vi "x502_recv.vi"() -> ()   [LabVIEW 2010]
uses:
  <vilib>/Waveform/DWDTOps.llb/DWDT Binary U32 to Digital.vi
panel:
  in  "Подключение по IP":bool
  in  "IP Addr":string="192.168.0.1"
  out "MCU ver":string
  in  "START":bool
  in  "Список устройств USB/PCIe":u16(ring) items=["L502, 111"]
  out "Mixed Signal Graph":T1(graph)
  in  "Логические каналы":T2(array[cluster])=[{"PhyCh"=1, "Avg"=1, "Mode"=1, "Range"=0}, {"PhyCh"=2, "Avg"=1, "Mode"=1, "Range"=0}, {"PhyCh"=3, "Avg"=1, "Mode"=1, "Range"=0}] {"Range" items=["10 В", "5 В", "2 В", "1 В", "0.5 В", "0.2 В"]; "Mode" items=["С общей землей", "Дифференциальный", "Измерение нуля"]; "Avg" max=255 step=1; "PhyCh" min=1 max=32 step=1}
  in  "Отображать за время":dbl=250.0 min=10.0 step=1.0
  in  "stop":bool
  out "Установленная частота синхронного ввода DIN":dbl=2.0 min=2.0 max=2000000.0 format="%#_8f"
  in  "Частота синхронного ввода DIN":dbl=20000.0 min=1.0 max=2000000.0 format="%#_8f"
  out "FPGA Ver":string
  in  "Количество каналов":u32=3 min=1 max=3
  out "Установленная частота на канал":dbl=2.0 min=2.0 max=2000000.0 format="%#_8f"
  out "Установленная частота сбора":dbl=2.0 min=2.0 max=2000000.0 format="%#_8f"
  in  "Частота сбора на канал":dbl=2000000.0 min=2.0 max=2000000.0 format="%#_8f"
  in  "Частота сбора (Гц)":dbl=2000000.0 min=2.0 max=2000000.0 format="%#_8f"
  out "PldaVer":u8
  out "Serial":string
  out "Name":string
  # "Информация о плате"
  # "Настройки модуля"
  # "Устанавливаемое"
  # "Установленное"
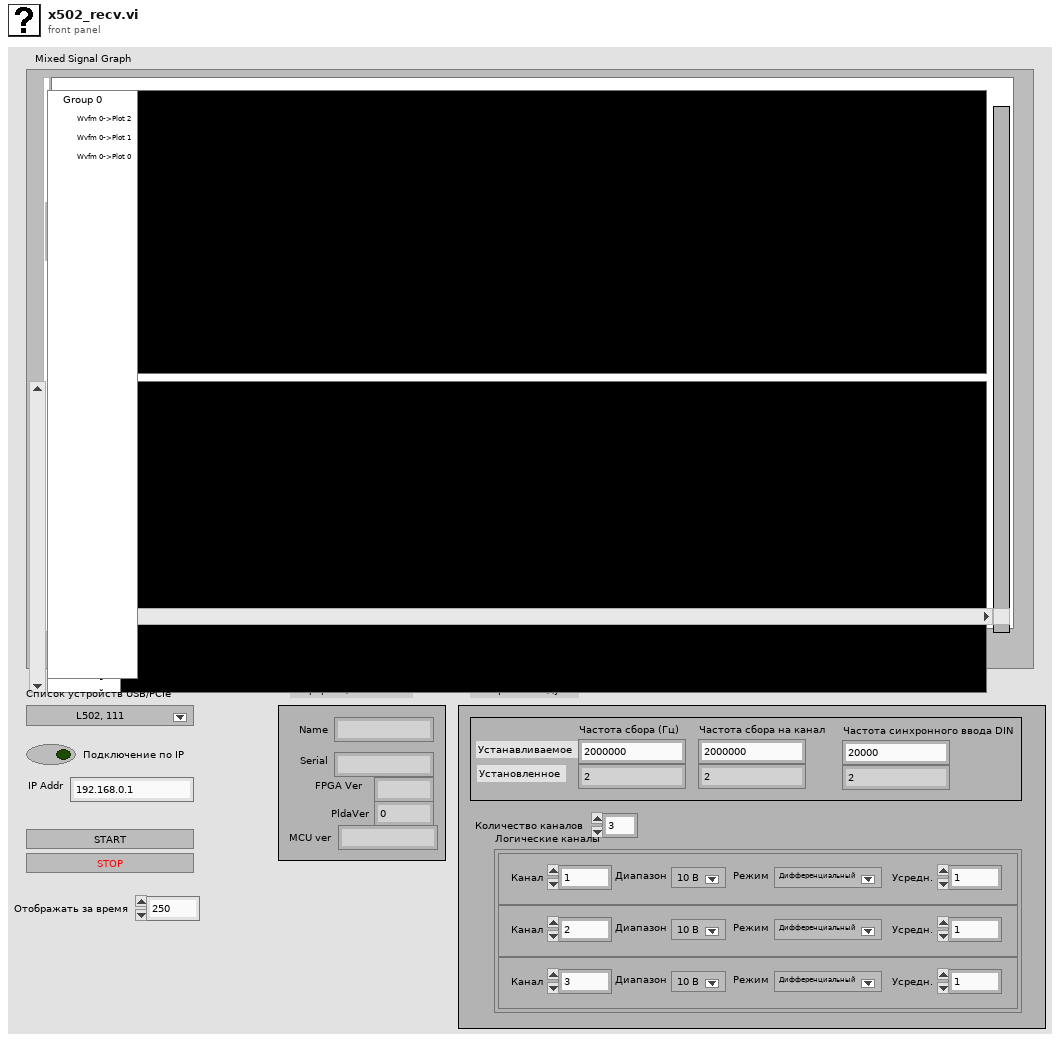
[diagram p1: front panel]
types:
  T1 = cluster{"Dynamic Data Type":dynamicdata, "digital waveform":digitalwaveform}
  T2 = cluster{"PhyCh":u32, "Avg":u32, "Mode":u32, "Range":u32}[]
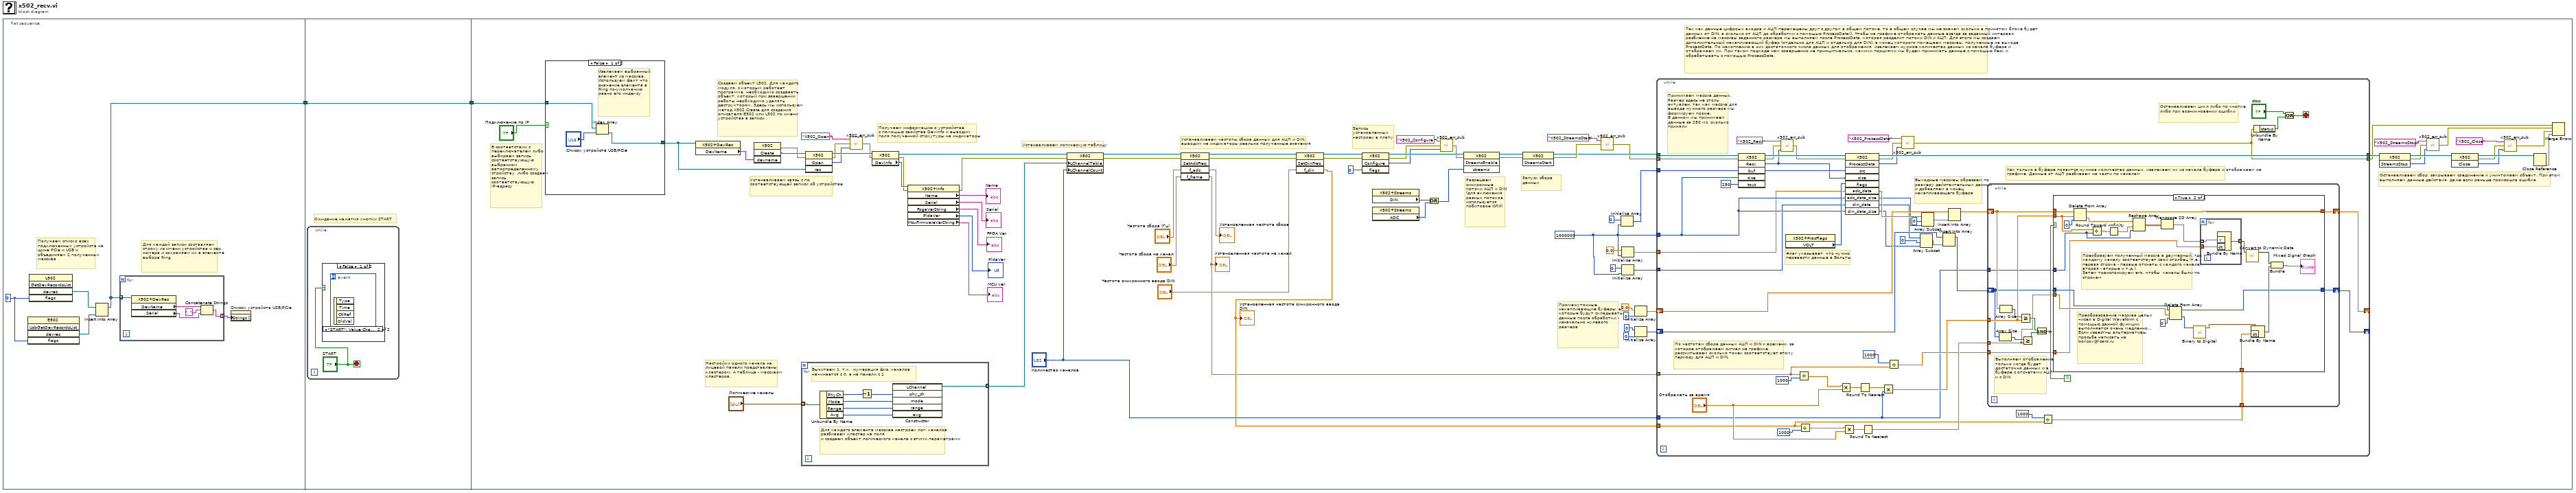
[diagram p0: block diagram]
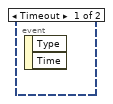
[diagram p2: hidden frame]
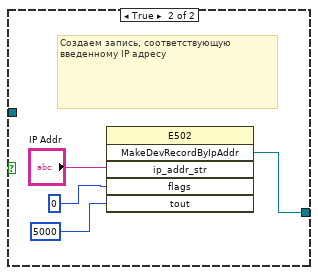
[diagram p4: hidden frame]
diagram:
  n1 = flat-sequence {
    tunnel: [w3] -> w1
    tunnel: [w13] -> w2
    tunnel: w1 -> [w13]
    tunnel: w2 -> [w21]
    frame #0 {
      w5 = 0
      # "Для каждой записи составляем строку из имени устройства и сер. номера и сохраняем их в элементе выбора Ring"
      # "Получаем списко всех подключенных устройств на шине PCIe и USB и объединяем 2 полученных массива"
      n2 = invoke class="E502" method="UsbGetDevRecordsList"("flags"=w5) -> ("devrec"=w6:refnum<k24>[])  [unwired: 4 in, 4 out]
      n3 = invoke class="L502" method="GetDevRecordsList"("flags"=w5) -> ("devrec"=w7:refnum<k24>[])  [unwired: 4 in, 4 out]
      n4 = Insert Into Array(array=w7, new element=w6) -> (w3:refnum<k24>[])  [unwired: 1 in]
      n5 = for {
        tunnel: [w9] -> w4 mode=indexing
        tunnel: w3 -> [w8] mode=indexing
        n6 = property class="X502+DevRec"(reference=w8) -> ("DevName"=w12:string, "Serial"=w10:string)  [unwired: 1 in, 2 out]
        n7 = Concatenate Strings(w12, ", ", w10) -> (w9:string)
      }
      n8 = property on="Список устройств USB/PCIe" class="Ring (strict)"("Strings []"=w4) -> ()  [unwired: 2 in, 2 out]
    }
    frame #1 {
      # "Ожидание нажатия кнопки START"
      n9 = while {
        stop <- "START" stop-if-true
        n10 = case shown="False" "START" {
          frame False {
            n11 = event shown="[1] \"START\": Value Change" {
              selector: _ -> [_ _]
              dyn-events: _ -> [_ _]
              timeout: _ -> [_ _]
              event Timeout {
                n12 = event-data() -> ()  [unwired: 1 in, 2 out]
              }
              event "START": Value Change {
                n13 = event-data() -> ()  [unwired: 1 in, 4 out]
              }
            }
          }
          frame True {
          }
        }
      }
    }
    frame #2 {
      w84 = u32 1000000 ("element")
      # "В соответствии с переключателем либо выбираем запись, соответствующую выбранном автоопределенному стройству, либо создаем запись, соответствующую IP-адресу"
      # "Останавливаем сбор, закрываем соединение и уничтожаем объект. При этом выполняем данные действия, даже если раньше произошла ошибка"
      # "Так как данные цифроых входов и АЦП перемешены друг с другом в общем потоке, то в общем случае мы не значем сколько в принятом блоке будет данных от DIN, а сколько от АЦП до обработки с помощью ProcessData(). Чтобы на графике отображать данные всегда за заданный интервал, разбиение на массивы заданного размера мы выполняем после ProcessData, которая разделит потоки DIN и АЦП. Для этого мы создаем дополнительный накапливающий буфер (отдельно для АЦП и отдельно для DIN), в конец которого помещаем массивы, полученные на выходе ProcessData. По накоплению в них достаточного числа данных для отображения  извлекаем нужное количество данных из начала буфера и отображаем их. При таком подходе нам совершенно не принципиально, какими порциями мы будем принимать данные с помощью Recv и обрабатывать с помощью ProcessData."
      # "Промежуточные накапливающие буферы, в которые будут складываться данные после обработки - изначально нулевого размера"
      # "Запуск сбора данных"
      # "Разрешаем синхронные потоки АЦП и DIN (для включения разных потоков используется побитовое ИЛИ)"
      # "Запись установленных настроек в плату"
      # "Устанавливаем частоты сбора данных для АЦП и DIN,\nвыводим на индикаторы реально полученные значения"
      # "Устанавливаем логическую таблицу"
      # "Настройки одного канала на лицевой панели представлены кластером. А таблица - массивом кластеров."
      # "Создаем объект L502. Для каждого модуля, с которым работает программа, необходимо создавать объект, который при завершении работы необходимо удалять деструктором. Здесь мы используем метод X502.Create для создания описателя E502 или L502 по имени устройства в записи"
      # "Получаем информацию о устройстве \nс помощью свойства DevInfo и выводим\nполя полученной стркутуры на индикаторы"
      # "Устанавливаем связь с по соответствующей записи об устройстве"
      n14 = case shown="False" "Подключение по IP" {
        tunnel: w21 -> [w93 _]
        tunnel: [w91 w94] -> w20
        frame False {
          # "Извлекаем выбранный элемент из массива. Используем факт что значение элемента в Ring по-умолчанию равно его индексу"
          n15 = Index Array(array=w93, index="Список устройств USB/PCIe") -> (element=w91:refnum<k24>)
        }
        frame True {
          # "Создаем запись, соответствующую введенному IP адресу"
          n16 = invoke class="E502" method="MakeDevRecordByIpAddr"("ip_addr_str"="IP Addr", "flags"=0, "tout"=5000) -> ("MakeDevRecordByIpAddr"=w94:refnum<k24>)  [unwired: 3 in, 5 out]
        }
      }
      n17 = property class="X502+DevRec"(reference=w20) -> ("DevName"=w52:string)  [unwired: 1 in, 2 out]
      n18 = invoke class="X502" method="Create"("devname"=w52) -> (error out=w51:errorcluster, "Create"=w53:refnum<k24>)  [unwired: 3 in, 2 out]
      n19 = for {
        tunnel: "Логические каналы" -> [w198] mode=indexing
        tunnel: [w192] -> w78 mode=indexing
        # "Вычитаем 1, т.к.  нумерация физ. каналов начинается с 0, а на панели с 1"
        # "Для каждого элемента массива настроек лог. каналов разбиваем кластер на поля\nи создаем объект логического канала с этими параметрами"
        n20 = Unbundle By Name(w198) -> ("PhyCh"=w197:u32, "Mode"=w195:u32, "Range"=w194:u32, "Avg"=w193:u32)
        n21 = Decrement(x=w197) -> (x-1=w196:u32)
        n22 = constructor class="X502+LChannel"("phy_ch"=w196, "mode"=w195, "range"=w194, "avg"=w193) -> (reference out=w192:refnum<k24>)  [unwired: 3 in, 6 out]
      }
      n23 = invoke class="X502" method="Open"(reference=w53, error in=w51, "rec"=w20) -> (reference out=w56:refnum<k24>, error out=w49:errorcluster, "Open"=w50:i32)  [unwired: 1 in, 1 out]
      n24 = call "x502_err_sub.vi"("Error code"=w50, "error in (no error)"=w49, "Error descr"="X502_Open ") -> ("error out"=w47:errorcluster)
      n25 = property class="X502"(reference=w56, error in=w47) -> (reference out=w57:refnum<k24>, error out=w45:errorcluster, "DevInfo"=w46:refnum<k24>)
      n26 = property class="X502+Info"(reference=w46, error in=w45) -> (error out=w22:errorcluster, "Name"=→"Name":string, "Serial"=→"Serial":string, "FpgaVerString"=→"FPGA Ver":string, "PldaVer"=→"PldaVer":u8, "McuFirmwareVerString"=→"MCU ver":string)  [unwired: 1 out]
      n27 = property class="X502"(reference=w57, error in=w22, "LChannelTable"=w78, "LChannelCount"="Количество каналов") -> (reference out=w58:refnum<k24>, error out=w59:errorcluster)
      n28 = invoke class="X502" method="SetAdcFreq"(reference=w58, error in=w59, "f_adc"="Частота сбора (Гц)", "f_frame"="Частота сбора на канал") -> (reference out=w63:refnum<k24>, error out=w64:errorcluster, "f_adc"=→"Установленная частота сбора":dbl, "f_frame"=w81:dbl)  [unwired: 1 in, 1 out]
      "Установленная частота на канал" <- w81
      n29 = invoke class="X502" method="SetDinFreq"(reference=w63, error in=w64, "f_din"="Частота синхронного ввода DIN") -> (reference out=w68:refnum<k24>, error out=w69:errorcluster, "f_din"=w82:dbl)  [unwired: 1 in, 1 out]
      "Установленная частота синхронного ввода DIN" <- w82
      n30 = invoke class="X502" method="Configure"(reference=w68, error in=w69, "flags"=0) -> (reference out=w70:refnum<k24>, error out=w39:errorcluster, "Configure"=w37:i32)  [unwired: 1 in, 1 out]
      n31 = property class="X502+Streams"() -> ("DIN"=w31:u32)  [unwired: 2 in, 2 out]
      n32 = property class="X502+Streams"() -> ("ADC"=w67:u32)  [unwired: 2 in, 2 out]
      n33 = Or(x=w31, y=w67) -> (x .or. y?=w30:u32)
      n34 = call "x502_err_sub.vi"("Error code"=w37, "error in (no error)"=w39, "Error descr"="X502_Configure ") -> ("error out"=w38:errorcluster)
      n35 = invoke class="X502" method="StreamsEnable"(reference=w70, error in=w38, "streams"=w30) -> (reference out=w71:refnum<k24>, error out=w72:errorcluster)  [unwired: 1 in, 2 out]
      n36 = invoke class="X502" method="StreamsStart"(reference=w71, error in=w72) -> (reference out=w33:refnum<k24>, error out=w35:errorcluster)  [unwired: 1 in, 1 out]
      n37 = call "x502_err_sub.vi"("error in (no error)"=w35, "Error descr"="X502_StreamsStart") -> ("error out"=w32:errorcluster)  [unwired: 1 in]
      n38 = Initialize Array(u32 0 ("element"), w84) -> (w85:u32[])
      n39 = Initialize Array(0.0 ("element"), w84) -> (w87:dbl[])
      n40 = Initialize Array(u32 0 ("element"), w84) -> (w86:u32[])
      n41 = Initialize Array(0.0 ("element"), u32 0 ("element")) -> (w89:dbl[])
      n42 = Initialize Array(u32 0 ("element"), u32 0 ("element")) -> (w88:u32[])
      n43 = while {
        tunnel: w33 -> [w150]
        tunnel: w32 -> [w149]
        tunnel: [w148] -> w29
        tunnel: w85 -> [w147]
        shift-right: [w142] -> _
        shift-left: w89 -> [w141]
        shift-right: [w113] -> _
        shift-left: w88 -> [w131]
        tunnel: "Количество каналов" -> [w98]
        tunnel: w81 -> [w114]
        tunnel: w82 -> [w116]
        tunnel: w84 -> [w112]
        tunnel: w86 -> [w111]
        tunnel: w87 -> [w110]
        tunnel: [w99] -> w15
        stop <- w119 stop-if-true
        # "Останавливаем цикл либо по кнопке, либо при возникновении ошибки"
        # "Как только в буфере появится нужное количество данных, извлекаем их из начала буфера и отображаем на графике. Данные от АЦП разбиваем на части по каналам"
        # "По частотам сбора данных АЦП и DIN и времени, за которое отображаем сигнал на графике, рассчитываем сколько точек соответствует этому периоду для АЦП и DIN."
        # "Выходные массивы обрезаем по размеру действительных данных и добавляем в конец накапливающего буфера"
        # "Флаг указывает, что нужно перевести данные в Вольты"
        # "Принимаем массив данных.\nРазмер здесь не столь актуален, так как массив для вывода нужного размера мы формируем позже.\nВ данном мы принимаем данные за 250 мс, сколько приняли"
        n44 = invoke class="X502" method="Recv"(reference=w150, error in=w149, "buf"=w147, "size"=w112, "tout"=u32 250 ("element")) -> (reference out=w138:refnum<k24>, error out=w106:errorcluster, "Recv"=w105:i32, "buf"=w146:u32[])  [unwired: 1 in, 2 out]
        n45 = call "x502_err_sub.vi"("Error code"=w105, "error in (no error)"=w106, "Error descr"="X502_Recv") -> ("error out"=w104:errorcluster)
        n46 = property class="X502+ProcFlags"() -> ("VOLT"=w137:u32)  [unwired: 2 in, 2 out]
        n47 = Divide(x=w114, y=1000) -> (x/y=w129:dbl)
        n48 = Divide(x=w116, y=1000) -> (x/y=w125:dbl)
        n49 = Multiply(x=w129, y="Отображать за время") -> (x*y=w128:dbl)
        n50 = Multiply(x=w125, y="Отображать за время") -> (x*y=w124:dbl)
        n51 = invoke class="X502" method="ProcessData"(reference=w138, error in=w104, "src"=w146, "size"=w105, "flags"=w137, "adc_data"=w110, "adc_data_size"=w112, "din_data"=w111, "din_data_size"=w112) -> (reference out=w148:refnum<k24>, error out=w102:errorcluster, "ProcessData"=w101:i32, "adc_data"=w144:dbl[], "adc_data_size"=w139:u32, "din_data"=w134:u32[], "din_data_size"=w133:u32)  [unwired: 1 in, 3 out]
        n52 = Round To Nearest(number=w128) -> (nearest integer value=w127:dbl)
        n53 = Round To Nearest(number=w124) -> (nearest integer value=w120:dbl)
        n54 = Multiply(x=w127, y=w98) -> (x*y=w121:dbl)
        n55 = Divide(x=u32 1000 ("element"), y=w114) -> (x/y=w109:dbl)
        n56 = call "x502_err_sub.vi"("Error code"=w101, "error in (no error)"=w102, "Error descr"="X502_ProcessData") -> ("error out"=w99:errorcluster)
        n57 = Array Subset(array=w134, index=u32 0 ("element"), length=w133) -> (w132:u32[])
        n58 = Array Subset(array=w144, index=u32 0 ("element"), length=w139) -> (w136:dbl[])
        n59 = Insert Into Array(array=w131, new element=w132) -> (w122:u32[])  [unwired: 1 in]
        n60 = Insert Into Array(array=w141, new element=w136) -> (w140:dbl[])  [unwired: 1 in]
        n61 = Divide(x=u32 1000 ("element"), y=w116) -> (x/y=w108:dbl)
        n62 = while {
          shift-right: [w164] -> w142
          shift-left: w140 -> [w163]
          shift-right: [w154] -> w113
          shift-left: w122 -> [w156]
          tunnel: w121 -> [w161]
          tunnel: w120 -> [w155]
          tunnel: w109 -> [w153]
          tunnel: w108 -> [w152]
          tunnel: w98 -> [w151]
          stop <- w157 continue-if-true
          # "Выполняем отображение только когда будет достаточно данных и в буфере с отсчетами АЦП и с DIN"
          n63 = Array Size(array=w156) -> (size(s)=w160:i32)
          n64 = Array Size(array=w163) -> (size(s)=w162:i32)
          n65 = Greater Or Equal?(x=w162, y=w161) -> (x >= y?=w158:bool)
          n66 = Greater Or Equal?(x=w160, y=w155) -> (x >= y?=w159:bool)
          n67 = And(x=w158, y=w159) -> (x .and. y?=w157:bool)
          n68 = case shown="True" w157 {
            tunnel: [w166 w188] -> w164
            tunnel: w163 -> [w166 w187]
            tunnel: w161 -> [_ w172]
            tunnel: w156 -> [w165 w178]
            tunnel: w155 -> [_ w177]
            tunnel: [w165 w182] -> w154
            tunnel: w153 -> [_ w170]
            tunnel: w152 -> [_ w180]
            tunnel: w151 -> [_ w167]
            frame False {
            }
            frame True {
              # "Преобразуем полученный массив в двумерный, где каждому каналу соответствует свой столбец (т.е. первая строка - первые отсчеты с каждого канала, вторая - вторые и т.д.).\nЗатем транспонируем его, чтобы  каналы были по строкам"
              # "Преобразование массива целых чисел в Digital Waveform с помощью данной функции выполняется очень медленно... Если известны альтернативы, просьба написать на borisov@lcard.ru"
              n69 = Delete From Array(array=w187, length=w172, index=u32 0 ("element")) -> (deleted portion=w171:dbl[], array with subset deleted=w188:dbl[])
              n70 = Divide(x=w172, y=w167) -> (x/y=w176:dbl)
              n71 = Round Toward -Infinity(1:w176) -> (0:w173:dbl)
              n72 = Reshape Array(w171, w173, w167) -> (w175:dbl[][])
              n73 = Transpose 2D Array(2D array=w175) -> (transposed array=w174:dbl[][])
              n74 = Delete From Array(array=w178, length=w177, index=u32 0 ("element")) -> (deleted portion=w184:u32[], array with subset deleted=w182:u32[])
              n75 = call-poly <vilib>:"Binary to Digital.vi"("binary array"=w184) -> ("digital waveform"=w179:digitalwaveform)  [unwired: 9 in, 1 out]
              n76 = for {
                tunnel: w174 -> [w190] mode=indexing
                tunnel: w170 -> [w191]
                tunnel: [w189] -> w169 mode=indexing
                n77 = Bundle By Name("Y"=w190, "dt"=w191) -> (w189:waveform(dbl))  [unwired: 1 in]
              }
              n78 = call "Convert to Dynamic Data"("Array of Waveforms"=w169) -> ("Dynamic Data Type"=w168:dynamicdata)  [unwired: 3 out]
              n79 = Bundle By Name(cluster=w179, "dt"=w180) -> (w183:digitalwaveform)
              n80 = Bundle("Dynamic Data Type"=w168, "digital waveform"=w183) -> (→"Mixed Signal Graph":T1)  [unwired: 1 in]
            }
          }
        }
        n81 = Unbundle By Name(w99) -> ("status"=w100:bool)
        n82 = Or(x="stop", y=w100) -> (x .or. y?=w119:bool)
      }
      n83 = invoke class="X502" method="StreamsStop"(reference=w29) -> (reference out=w54:refnum<k24>, error out=w28:errorcluster, "StreamsStop"=w26:i32)  [unwired: 2 in]
      n84 = call "x502_err_sub.vi"("Error code"=w26, "error in (no error)"=w28, "Error descr"="X502_StreamsStop") -> ("error out"=w16:errorcluster)
      n85 = invoke class="X502" method="Close"(reference=w54) -> (reference out=w55:refnum<k24>, error out=w24:errorcluster, "Close"=w23:i32)  [unwired: 2 in]
      n86 = call "x502_err_sub.vi"("Error code"=w23, "error in (no error)"=w24, "Error descr"="X502_Close") -> ("error out"=w17:errorcluster)
      n87 = Close Reference(reference=w55) -> (error out=w18:errorcluster)  [unwired: 1 in]
      n88 = Merge Errors(w15, w16, w17, w18) -> ()  [unwired: 1 out]
    }
  }
